vi "SPD.DT Meas.vi"(5 "Progress":refnum<vi>, 7 "Continue":refnum<vi>, 8 "Error In":errorcluster, 11 "SPD.Stand Ctrl in":T1={"spdDeviceSession"={"spdRef"=0, "connected"=FALSE, "spdName"="", "specification"={"diod case"=enum."default", "type"=enum."Unknown", "frequency"=enum."Unknown"}, "hidSPD.Controller"={"TSet"=0.0, "HV_bias"=0.0, "DDS_stb_code"=0}, "hidSPD.Sturtup Values"={"TSet"=0.0, "HV_bias"=0.0, "DDS_stb_code"=0}}, "DevBSession"={"DevBRef"="", "connected"=FALSE}, "FreqCSession"={"FreqCRef"="", "timeout"=0.0, "Gate"=0.0, "connected"=FALSE}, "8164BSession"={"Connection ID"=refnum, "Connected"=FALSE, "Info"="", "Slots Info"=[]}, "LeCroySession"={"LeCroySession"="", "connected"=FALSE}, "Events"={"DCRTest"=refnum, "Stop"=refnum}, "configFile"={"configFile ref"=refnum, "configFile path"=path "", "equipmentFile ref"=refnum}, "SPD.Meas Grid"={"DateTime"="", "DT"=[], "Insensitivity"=[], "Temprature"=[], "Stb_code"=[], "HV_Bias"=[]}, "SPD.Queues"={"state queue"=refnum}, "Console"=refnum} {"spdDeviceSession"."hidSPD.Sturtup Values"."HV_bias" format="%#_6p, V"; "spdDeviceSession"."hidSPD.Sturtup Values"."TSet" format="%#_6p, DegC"; "spdDeviceSession"."hidSPD.Controller"."HV_bias" format="%#_6p, V"; "spdDeviceSession"."hidSPD.Controller"."TSet" format="%#_6p, DegC"}) -> (0 "Error Out":errorcluster, 1 "pass":bool, 2 "Report":string, 3 "SPD.Stand Ctrl out":T1={"spdDeviceSession"={"spdRef"=0, "connected"=FALSE, "spdName"="", "specification"={"diod case"=enum."default", "type"=enum."Unknown", "frequency"=enum."Unknown"}, "hidSPD.Controller"={"TSet"=0.0, "HV_bias"=0.0, "DDS_stb_code"=0}, "hidSPD.Sturtup Values"={"TSet"=0.0, "HV_bias"=0.0, "DDS_stb_code"=0}}, "DevBSession"={"DevBRef"="", "connected"=FALSE}, "FreqCSession"={"FreqCRef"="", "timeout"=0.0, "Gate"=0.0, "connected"=FALSE}, "8164BSession"={"Connection ID"=refnum, "Connected"=FALSE, "Info"="", "Slots Info"=[]}, "LeCroySession"={"LeCroySession"="", "connected"=FALSE}, "Events"={"DCRTest"=refnum, "Stop"=refnum}, "configFile"={"configFile ref"=refnum, "configFile path"=path "", "equipmentFile ref"=refnum}, "SPD.Meas Grid"={"DateTime"="", "DT"=[], "Insensitivity"=[], "Temprature"=[], "Stb_code"=[], "HV_Bias"=[]}, "SPD.Queues"={"state queue"=refnum}, "Console"=refnum} {"spdDeviceSession"."hidSPD.Sturtup Values"."HV_bias" format="%#_6p, V"; "spdDeviceSession"."hidSPD.Sturtup Values"."TSet" format="%#_6p, DegC"; "spdDeviceSession"."hidSPD.Controller"."HV_bias" format="%#_6p, V"; "spdDeviceSession"."hidSPD.Controller"."TSet" format="%#_6p, DegC"})   [LabVIEW 2018]
uses:
  typedefs/SPD.Stand Ctrl.ctl
  Instruments/SPD HID Interface/hidSPDLibForLabView/LibVIs/hidSPD Controls/hidSPD Device Session.ctl
  Instruments/SPD HID Interface/hidSPDLibForLabView/LibVIs/hidSPD Controls/hidSPD.SPD specification.ctl
  Instruments/SPD HID Interface/hidSPDLibForLabView/LibVIs/hidSPD Controls/hidSPD SPD Diod Case.ctl
  Instruments/SPD HID Interface/hidSPDLibForLabView/LibVIs/hidSPD Controls/hidSPD SPD Type.ctl
  Instruments/SPD HID Interface/hidSPDLibForLabView/LibVIs/hidSPD Controls/hidSPD.STB Frequency.ctl
  Instruments/SPD HID Interface/hidSPDLibForLabView/LibVIs/hidSPD Controls/hidSPD Controller.ctl
  Instruments/KC705 DevBoard/typedefs/DevB.Session.ctl
  Instruments/KeySight 53230A/typedefs/FreqC.Session.ctl
  Instruments/KeySight 8164B/KeySight 8164B LAN InstrLib/typedefs/KeySight 8164B control.ctl
  Instruments/LeCroy SDA830/typedefs/LeCroy.Session.ctl
  typedefs/SPD.Events.ctl
  ConfigFile/SPD.Config File ctrl.ctl
  <vilib>/Utility/config.llb/Config Data RefNum.ctl
  typedefs/SPD.Meas Grid.ctl
  typedefs/SPD.Queues.ctl
  typedefs/SPD.Stand state.ctl
  Instruments/KeySight 8164B/KeySight 8164B LAN InstrLib.lvlib
  <vilib>/Utility/config.llb/NI_LVConfig.lvlib
  Instruments/SPD HID Interface/hidSPDLibForLabView/hidSPDLibForLabView.lvlib
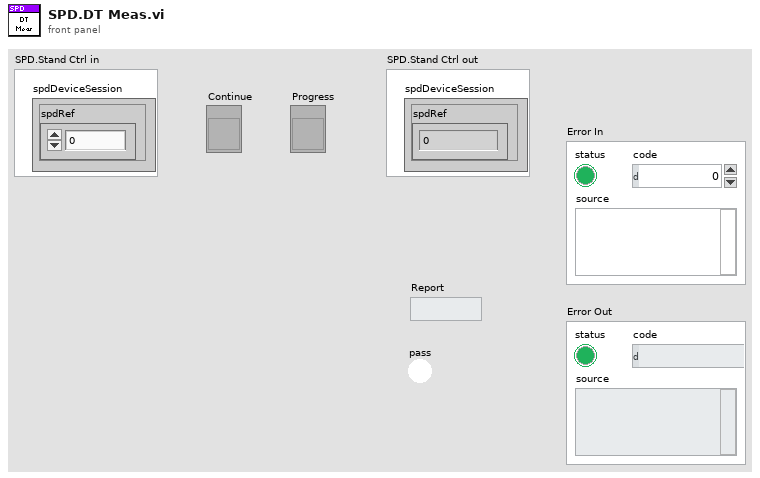
[diagram p1: front panel]
types:
  T1 = typedef "SPD.Stand Ctrl.ctl" = cluster{"spdDeviceSession":T2, "DevBSession":T8, "FreqCSession":T9, "8164BSession":T10, "LeCroySession":T11, "Events":T12, "configFile":T13, "SPD.Meas Grid":T15, "SPD.Queues":T16, "Console":refnum<vi>}
  T2 = typedef "hidSPDLibForLabView.lvlib/hidSPD Device Session.ctl" = cluster{"spdRef":u64, "connected":bool, "spdName":string, "specification":T3, "hidSPD.Controller":T7, "hidSPD.Sturtup Values":T7}
  T3 = typedef "hidSPDLibForLabView.lvlib/hidSPD.SPD specification.ctl" = cluster{"diod case":T4, "type":T5, "frequency":T6}
  T4 = typedef "hidSPDLibForLabView.lvlib/hidSPD SPD Diod Case.ctl" = enum16{"Unknown", "default", "butterfly"}
  T5 = typedef "hidSPDLibForLabView.lvlib/hidSPD SPD Type.ctl" = enum16{"Unknown", "Free Run", "Gate"}
  T6 = typedef "hidSPDLibForLabView.lvlib/hidSPD.STB Frequency.ctl" = enum16{"Unknown", "312", "1250"}
  T7 = typedef "hidSPDLibForLabView.lvlib/hidSPD Controller.ctl" = cluster{"TSet":sgl, "HV_bias":sgl, "DDS_stb_code":u16}
  T8 = typedef "DevB.Session.ctl" = cluster{"DevBRef":refnum<visa-resource-name>, "connected":bool}
  T9 = typedef "FreqC.Session.ctl" = cluster{"FreqCRef":refnum<visa-resource-name>, "timeout":dbl, "Gate":dbl, "connected":bool}
  T10 = typedef "KeySight 8164B LAN InstrLib.lvlib/KeySight 8164B control.ctl" = cluster{"Connection ID":refnum<k5>, "Connected":bool, "Info":string, "Slots Info":string[]}
  T11 = typedef "LeCroy.Session.ctl" = cluster{"LeCroySession":refnum<visa-resource-name>, "connected":bool}
  T12 = typedef "SPD.Events.ctl" = cluster{"DCRTest":refnum<user-event>, "Stop":refnum<user-event>}
  T13 = typedef "SPD.Config File ctrl.ctl" = cluster{"configFile ref":T14, "configFile path":path, "equipmentFile ref":T14}
  T14 = typedef "NI_LVConfig.lvlib/Config Data RefNum.ctl" = refnum<k1>
  T15 = typedef "SPD.Meas Grid.ctl" = cluster{"DateTime":string, "DT":dbl[], "Insensitivity":dbl[], "Temprature":dbl[], "Stb_code":dbl[], "HV_Bias":dbl[][][][]}
  T16 = typedef "SPD.Queues.ctl" = cluster{"state queue":refnum<queue>}
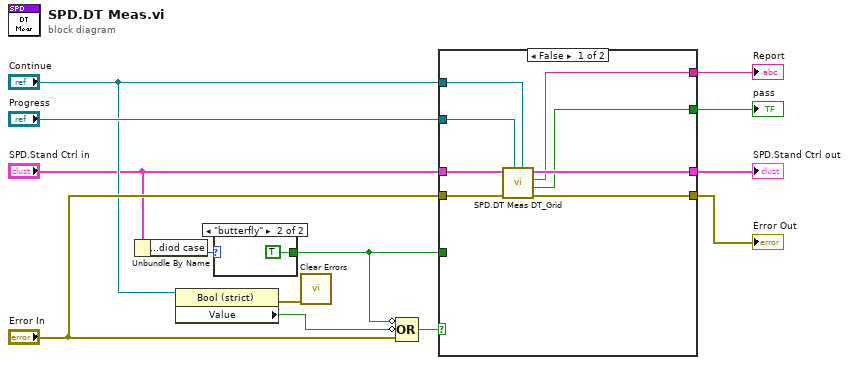
[diagram p0: block diagram]
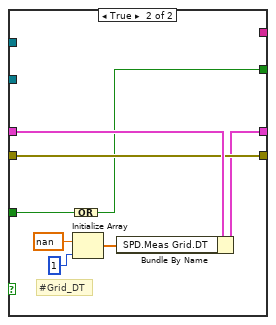
[diagram p3: hidden frame]
diagram:
  n1 = Unbundle By Name("SPD.Stand Ctrl in") -> ("spdDeviceSession.specification.diod case"=w2:T4)
  n2 = property class="Bool (strict)"(reference="Continue") -> (error out=w6:errorcluster, "Value"=w5:bool)  [unwired: 1 in, 1 out]
  n3 = case shown="\"butterfly\"" w2 {
    tunnel: [_ TRUE] -> w1
    frame "Unknown", Default {
    }
    frame "butterfly" {
    }
  }
  n4 = call <vilib>:"Clear Errors.vi"("error in (no error)"=w6) -> ()  [unwired: 5 in, 2 out]
  n5 = Compound Arithmetic op=OR(invert w1, invert w5, "Error In") -> (w8:bool)
  n6 = case shown="False" w8 {
    tunnel: [w22 w29] -> w13
    tunnel: "SPD.Stand Ctrl in" -> [w16 w30]
    tunnel: [w21 w26] -> w12
    tunnel: "Progress" -> [w20 _]
    tunnel: "Continue" -> [w19 _]
    tunnel: [w18 _] -> w10
    tunnel: [w17 w27] -> w9
    tunnel: "Error In" -> [w15 w29]
    tunnel: w1 -> [_ w28]
    frame False {
      n7 = call "SPD.DT Meas DT_Grid.vi"("Continue"=w19, "Progress"=w20, "Error In"=w15, "SPD.Stand Ctrl in"=w16) -> ("Error Out"=w22:errorcluster, "pass"=w17:bool, "Report"=w18:string, "SPD.Stand Ctrl out"=w21:T1)  [unwired: 4 in]
    }
    frame True {
      # "#Grid_DT"
      n8 = Initialize Array(nan ("element"), 1 ("dimension size")) -> (w23:dbl[])
      n9 = Compound Arithmetic op=OR(w28) -> (w27:bool)
      n10 = Bundle By Name(cluster=w30, "SPD.Meas Grid.DT"=w23) -> (w26:T1)
    }
  }
  "Error Out" <- w13
  "SPD.Stand Ctrl out" <- w12
  "Report" <- w10
  "pass" <- w9
